vi "select_data.vi"(7 "connection_reference":T1, 8 "error in (no error)":errorcluster, 10 "range_finish_utc":dbl format="%^<%H:%M:%S%4u %m/%d/%y>T", 11 "range_start_utc":dbl format="%^<%H:%M:%S%4u %m/%d/%y>T") -> (0 "error out":errorcluster, 3 "data_read":cluster{"time":dbl, "value":dbl}[](array[cluster]) {"value" format="%#_10f"; "time" format="%^<%H:%M:%S%3u %m/%d/%y>T"})   [LabVIEW 2015, in "lv-example-postgres.lvlib"]
uses:
  lv-example-postgres.lvlib
  <vilib>/addons/database/Connection.llb/Conn ObjectReference.ctl
  <vilib>/addons/database/Command.llb/Cmd Execute.vi
  <vilib>/addons/database/Recordset.llb/Rec Fetch Recordset Data (CR).vi
  <vilib>/addons/database/Recordset.llb/Rec Destroy - Command.vi
  <vilib>/addons/database/Command.llb/Cmd Delete.vi
  <vilib>/addons/database/NI_Database_API.lvlib
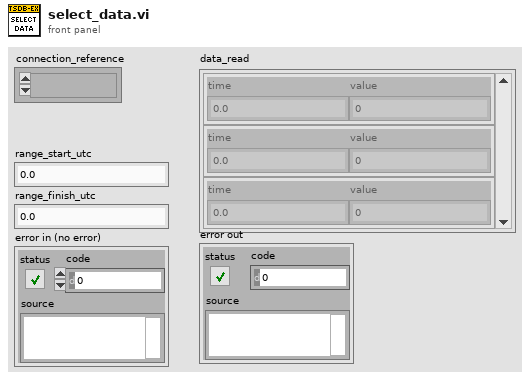
[diagram p1: front panel]
types:
  T1 = typedef "NI_Database_API.lvlib/Conn ObjectReference.ctl" = refnum<k1>
  T2 = typedef "NI_Database_API.lvlib/DB Tools Parameter Info.ctl" = cluster{"parameter name":string, "type":T3, "direction":T4, "value":variant}
  T3 = typedef "NI_Database_API.lvlib/DB Tools DataTypes.ctl" = enum16{"String", "Long (I32)", "Single (SGL)", "Double (DBL)", "Date/Time", "Binary"}
  T4 = typedef "NI_Database_API.lvlib/DB Tools Parameter Dir.ctl" = enum32{"Input", "Output", "Input/Output", "Return Value"}
  T5 = typedef "NI_Database_API.lvlib/Cmd ObjectReference.ctl" = refnum<k1>
  T6 = typedef "NI_Database_API.lvlib/Cmd-Rec Object Reference.ctl" = refnum<k1>
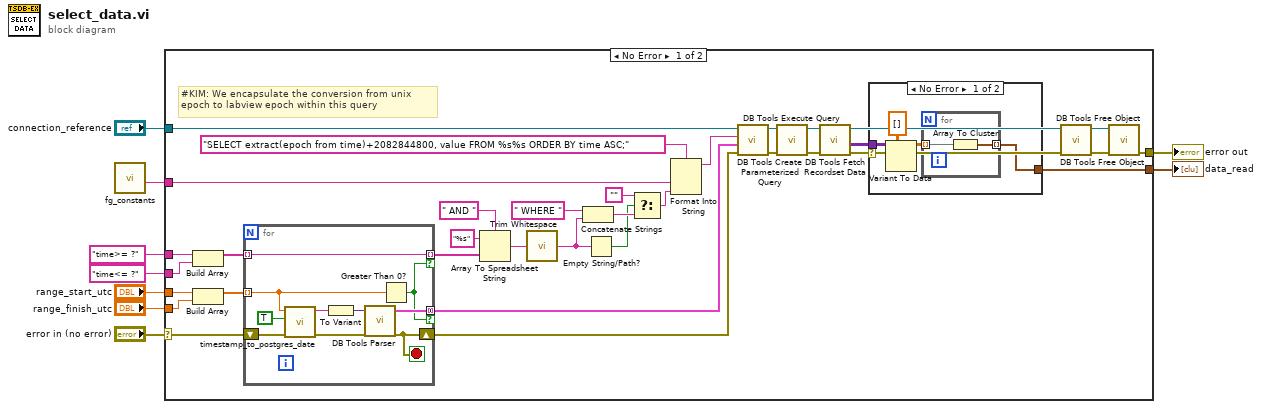
[diagram p0: block diagram]
diagram:
  n1 = call "fg_constants.vi"() -> ("table out"=w1:string)  [unwired: 9 in, 2 out]
  n2 = case shown="No Error" "error in (no error)" {
    selector: "error in (no error)" -> [w36 w60]
    tunnel: [w43 _] -> w9
    tunnel: w1 -> [w14 _]
    tunnel: "connection_reference" -> [w18 _]
    tunnel: [w11 w60] -> w6
    tunnel: "range_start_utc" -> [w38 _]
    tunnel: "range_finish_utc" -> [w37 _]
    tunnel: "time>= ?" ("format string") -> [w40 _]
    tunnel: "time<= ?" ("format string") -> [w39 _]
    frame No Error {
      # "#KIM: We encapsulate the conversion from unix\nepoch to labview epoch within this query"
      n3 = Build Array(w40, w39) -> (w35:string[])
      n4 = Build Array(w38, w37) -> (w30:dbl[])
      n5 = for {
        tunnel: w35 -> [w50] mode=indexing
        tunnel: w30 -> [w58] mode=indexing
        tunnel: [w50] -> w28 mode=indexing if=w51
        shift-right: [w54] -> w15
        shift-left: w36 -> [w59]
        tunnel: [w52] -> w13 mode=concatenating if=w51
        stop <- w54 stop-if-true
        n6 = call "timestamp_to_postgres_date.vi"("error in (no error)"=w59, "utc"=TRUE, "date_time"=w58) -> ("error out"=w55:errorcluster, "postgres_date"=w56:string)  [unwired: 7 in]
        n7 = To Variant(anything=w56) -> (Variant=w53:variant)
        n8 = call <vilib>:"DB Tools Parser.vi"("error in (no error)"=w55, "variant"=w53) -> ("error out"=w54:errorcluster, "parameters"=w52:T2[])  [unwired: 2 in]
        n9 = Greater Than 0?(x=w58) -> (x > 0?=w51:bool)
      }
      n10 = Array To Spreadsheet String(delimiter (Tab)=" AND " ("format string"), array=w28, 3:"%s" ("format string")) -> (spreadsheet string=w32:string)
      n11 = call <vilib>:"Trim Whitespace.vi"("string"=w32) -> ("trimmed string"=w26:string)  [unwired: 1 in]
      n12 = Concatenate Strings(" WHERE " ("format string"), w26) -> (w27:string)
      n13 = Empty String/Path?(string/path=w26) -> (empty?=w25:bool)
      n14 = Select(t="", s=w25, f=w27) -> (s? t:f=w16:string)
      n15 = Format Into String(format string="SELECT extract(epoch from time)+2082844800, value FROM %s%s ORDER BY time ASC;", w14, w16) -> (resulting string=w17:string)  [unwired: 2 in, 1 out]
      n16 = call <vilib>:"DB Tools Create Parameterized Query.vi"("error in (no error)"=w15, "parameters"=w13, "SQL query"=w17, "connection reference"=w18) -> ("error out"=w24:errorcluster, "command reference"=w23:T5)  [unwired: 3 in, 1 out]
      n17 = call-poly <vilib>:"DB Tools Execute Query.vi"("error in (no error)"=w24, "command reference"=w23) -> ("error out"=w21:errorcluster, "command-recordset reference"=w20:T6)  [unwired: 6 in]
      n18 = call-poly <vilib>:"DB Tools Fetch Recordset Data.vi"("error in (no error)"=w21, "command-recordset reference"=w20) -> ("error out"=w10:errorcluster, "recordset data"=w42:variant[][], "command-recordset reference out"=w19:T6)  [unwired: 3 in]
      n19 = case shown="No Error" w10 {
        tunnel: [w47 _] -> w43
        tunnel: w42 -> [w45 _]
        frame No Error {
          n20 = Variant To Data(type=dbl[][] [] ("Array"), Variant=w45) -> (data=w44:dbl[][])  [unwired: 1 in, 1 out]
          n21 = for {
            tunnel: w44 -> [w48] mode=indexing
            tunnel: [w49] -> w47 mode=indexing
            n22 = Array To Cluster(array=w48) -> (cluster=w49:cluster{"Array[0]":dbl, "Array[1]":dbl})
          }
        }
        frame Error {
        }
      }
      n23 = call-poly <vilib>:"DB Tools Free Object.vi"("error in (no error)"=w10, "command-recordset reference"=w19) -> ("error out"=w12:errorcluster, "command reference"=w22:T5)  [unwired: 8 in]
      n24 = call-poly <vilib>:"DB Tools Free Object.vi"("error in (no error)"=w12, "command reference"=w22) -> ("error out"=w11:errorcluster)  [unwired: 8 in, 1 out]
    }
    frame Error {
    }
  }
  "data_read" <- w9
  "error out" <- w6
